vi "movingaverage_sdl.vi"(2 "input array":dbl[](array[numeric]), 3 "new element":dbl) -> (0 "Array":dbl[](array[numeric]), 1 "avg":dbl)   [LabVIEW 2011]
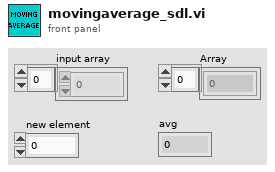
[diagram p1: front panel]
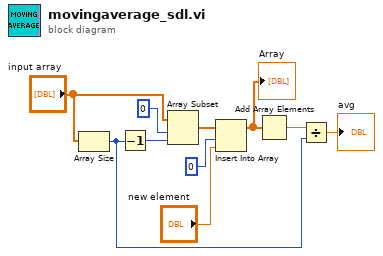
[diagram p0: block diagram]
diagram:
  n1 = Array Size(array="input array") -> (size(s)=w9:i32)
  n2 = Decrement(x=w9) -> (x-1=w5:i32)
  n3 = Array Subset(array="input array", index=0, length=w5) -> (w3:dbl[])
  n4 = Insert Into Array(array=w3, index=0, new element="new element") -> (w7:dbl[])
  "Array" <- w7
  n5 = Add Array Elements(numeric array=w7) -> (sum=w8:dbl)
  n6 = Divide(x=w8, y=w9) -> (x/y=→"avg":dbl)
